vi "MockSimpleGUI.vi"(11 "Controlling VI Path":path) -> ()   [LabVIEW 2022 SP3]
uses:
  <vilib>/Utility/miscctls.llb/LVRectTypeDef.ctl
panel:
  out "Front Panel Window:Window Bounds":T1
  in  "Option":bool
  out "Array":bool[](array[boolean])
  out "Execution:State":T2(ring)
  out "Status":string
  in  "Speed":dbl=3000.0
  out "Boolean":bool
  in  "GO Button":bool
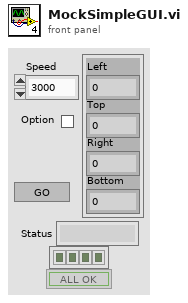
[diagram p1: front panel]
types:
  T1 = typedef "LVRectTypeDef.ctl" = cluster{"Left":i16, "Top":i16, "Right":i16, "Bottom":i16}
  T2 = enum32{"Bad", "Idle", "Run top level", "Running"}
  T3 = enum8{"Enabled", "Disabled", "Disabled and Grayed Out"}
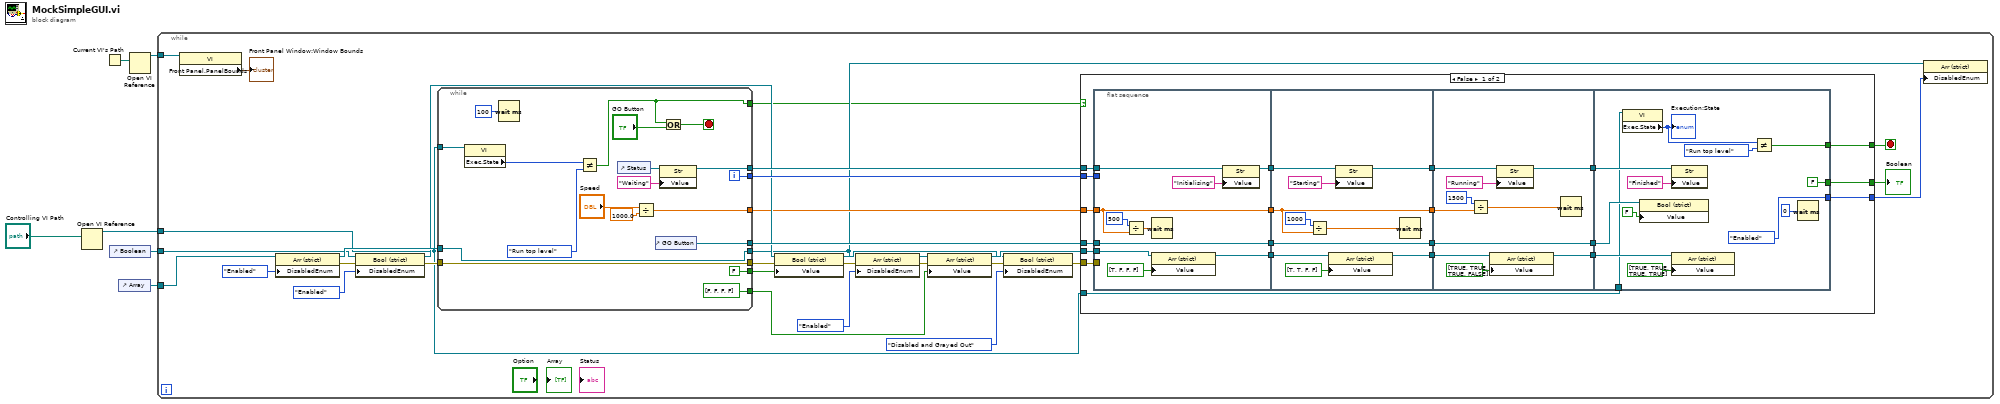
[diagram p0: block diagram]
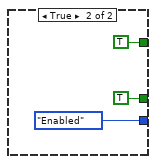
[diagram p2: hidden frame]
diagram:
  n1 = Open VI Reference(vi path="Controlling VI Path") -> (vi reference=w5:refnum<vi>)  [unwired: 5 in, 1 out]
  n2 = Current VI's Path() -> (path=w4:path)
  n3 = control-ref of="Boolean"() -> (w2:refnum<vi>)
  n4 = control-ref of="Array"() -> (w3:refnum<vi>)
  n5 = Open VI Reference(vi path=w4) -> (vi reference=w1:refnum<vi>)  [unwired: 5 in, 1 out]
  n6 = while {
    tunnel: w5 -> [w9]
    tunnel: w3 -> [w30]
    tunnel: w2 -> [w25]
    tunnel: w1 -> [w19]
    stop <- w8 stop-if-true
    n7 = property class="VI"(reference=w19) -> ("Front Panel.PanelBounds"=→"Front Panel Window:Window Bounds":T1)  [unwired: 1 in, 2 out]
    n8 = property class="Arr (strict)"(reference=w30, "DisabledEnum"=T3."Enabled" ("Disabled")) -> (reference out=w32:refnum<vi>, error out=w22:errorcluster)  [unwired: 1 in]
    n9 = property class="Bool (strict)"(reference=w25, error in=w22, "DisabledEnum"=T3."Enabled" ("Disabled")) -> (reference out=w24:refnum<vi>, error out=w23:errorcluster)
    n10 = while {
      tunnel: [w124] -> w38
      tunnel: [w117] -> w37
      tunnel: [bool[] [FALSE, FALSE, FALSE, FALSE] ("Array")] -> w35
      tunnel: [FALSE ("Value")] -> w29
      tunnel: [w120] -> w33
      tunnel: [w116] -> w17
      tunnel: w32 -> [w116]
      tunnel: w23 -> [w115]
      tunnel: [w115] -> w28
      tunnel: [w112] -> w18
      tunnel: w9 -> [w109]
      tunnel: [w106] -> w7
      i -> [w124]
      stop <- w107 stop-if-true
      n11 = property class="VI"(reference=w109) -> ("Exec.State"=w111:T2)  [unwired: 1 in, 2 out]
      n12 = Wait (ms)(milliseconds to wait=u32 100) -> ()  [unwired: 1 out]
      n13 = Not Equal?(x=w111, y=T2."Run top level" ("Execution:State")) -> (x != y?=w106:bool)
      n14 = control-ref of="Status"() -> (w119:refnum<vi>)
      n15 = Divide(x="Speed", y=1000.0) -> (x/y=w112:dbl)
      n16 = control-ref of="GO Button"() -> (w120:refnum<vi>)
      n17 = property class="Str"(reference=w119, "Value"="Waiting") -> (reference out=w117:refnum<vi>)  [unwired: 1 in, 1 out]
      n18 = Or(x=w106, y="GO Button") -> (x .or. y?=w107:bool)
    }
    n19 = property class="Bool (strict)"(reference=w24, error in=w28, "Value"=w29) -> (reference out=w21:refnum<vi>, error out=w27:errorcluster)
    n20 = property class="Arr (strict)"(reference=w17, error in=w27, "DisabledEnum"=T3."Enabled" ("Disabled")) -> (reference out=w31:refnum<vi>, error out=w26:errorcluster)
    n21 = property class="Arr (strict)"(reference=w31, error in=w26, "Value"=w35) -> (reference out=w34:refnum<vi>, error out=w13:errorcluster)
    n22 = property class="Bool (strict)"(reference=w21, error in=w13, "DisabledEnum"=T3."Disabled and Grayed Out" ("Disabled")) -> (error out=w12:errorcluster)  [unwired: 1 out]
    n23 = case shown="False" w7 {
      tunnel: w38 -> [w48 _]
      tunnel: w37 -> [w47 _]
      tunnel: [w46 TRUE] -> w36
      tunnel: w34 -> [w45 _]
      tunnel: w33 -> [w44 _]
      tunnel: w18 -> [w43 _]
      tunnel: [w42 T3."Enabled" ("Disabled")] -> w16
      tunnel: w12 -> [w41 _]
      tunnel: w9 -> [w40 _]
      tunnel: [w39 TRUE] -> w8
      frame False {
        n24 = flat-sequence {
          tunnel: w48 -> [_]
          tunnel: w47 -> [w69]
          tunnel: [w67] -> w59
          tunnel: w45 -> [w66]
          tunnel: [w64] -> w58
          tunnel: w44 -> [w63]
          tunnel: [w63] -> w57
          tunnel: w43 -> [w60]
          tunnel: [w60] -> w56
          tunnel: w41 -> [_]
          tunnel: w59 -> [w79]
          tunnel: [w77] -> w55
          tunnel: w58 -> [w75]
          tunnel: [w74] -> w54
          tunnel: [w73] -> w53
          tunnel: w57 -> [w73]
          tunnel: w56 -> [w70]
          tunnel: [w70] -> w52
          tunnel: w55 -> [w89]
          tunnel: [w88] -> w51
          tunnel: w54 -> [w86]
          tunnel: [w84] -> w50
          tunnel: [w83] -> w49
          tunnel: w53 -> [w83]
          tunnel: w52 -> [w82]
          tunnel: w51 -> [w102]
          tunnel: [FALSE] -> w46
          tunnel: w50 -> [w98]
          tunnel: w49 -> [w96]
          tunnel: [T3."Enabled" ("Disabled")] -> w42
          tunnel: w40 -> [w93]
          tunnel: [w90] -> w39
          frame #0 {
            n25 = Divide(x=u32 500 ("milliseconds to wait"), y=w60) -> (x/y=w61:dbl)
            n26 = Wait (ms)(milliseconds to wait=w61) -> ()  [unwired: 1 out]
            n27 = property class="Arr (strict)"(reference=w66, "Value"=bool[] [TRUE, FALSE, FALSE, FALSE] ("Array")) -> (reference out=w64:refnum<vi>)  [unwired: 1 in, 1 out]
            n28 = property class="Str"(reference=w69, "Value"="Initialising") -> (reference out=w67:refnum<vi>)  [unwired: 1 in, 1 out]
          }
          frame #1 {
            n29 = Divide(x=u32 1000 ("milliseconds to wait"), y=w70) -> (x/y=w71:dbl)
            n30 = property class="Arr (strict)"(reference=w75, "Value"=bool[] [TRUE, TRUE, FALSE, FALSE] ("Array")) -> (reference out=w74:refnum<vi>)  [unwired: 1 in, 1 out]
            n31 = property class="Str"(reference=w79, "Value"="Starting") -> (reference out=w77:refnum<vi>)  [unwired: 1 in, 1 out]
            n32 = Wait (ms)(milliseconds to wait=w71) -> ()  [unwired: 1 out]
          }
          frame #2 {
            n33 = Divide(x=u32 1500 ("milliseconds to wait"), y=w82) -> (x/y=w80:dbl)
            n34 = property class="Arr (strict)"(reference=w86, "Value"=bool[] [TRUE, TRUE, TRUE, FALSE] ("Array")) -> (reference out=w84:refnum<vi>)  [unwired: 1 in, 1 out]
            n35 = property class="Str"(reference=w89, "Value"="Running") -> (reference out=w88:refnum<vi>)  [unwired: 1 in, 1 out]
            n36 = Wait (ms)(milliseconds to wait=w80) -> ()  [unwired: 1 out]
          }
          frame #3 {
            n37 = property class="VI"(reference=w93) -> ("Exec.State"=w92:T2)  [unwired: 1 in, 2 out]
            "Execution:State" <- w92
            n38 = property class="Bool (strict)"(reference=w96, "Value"=FALSE) -> ()  [unwired: 1 in, 2 out]
            n39 = property class="Str"(reference=w102, "Value"="Finished") -> ()  [unwired: 1 in, 2 out]
            n40 = property class="Arr (strict)"(reference=w98, "Value"=bool[] [TRUE, TRUE, TRUE, TRUE] ("Array")) -> ()  [unwired: 1 in, 2 out]
            n41 = Not Equal?(x=w92, y=T2."Run top level" ("Execution:State")) -> (x != y?=w90:bool)
            n42 = Wait (ms)(milliseconds to wait=u32 0) -> ()  [unwired: 1 out]
          }
        }
      }
      frame True {
      }
    }
    "Boolean" <- w36
    n43 = property class="Arr (strict)"(reference=w17, "DisabledEnum"=w16) -> ()  [unwired: 1 in, 2 out]
  }
